vi "Set API Server.vi"(8 "error in (no error)":errorcluster, 11 "API Server":T1) -> (0 "error out":errorcluster)   [LabVIEW 2020, in "GCentral-API.lvlib"]
uses:
  GCentral-API.lvlib
  API Server.ctl
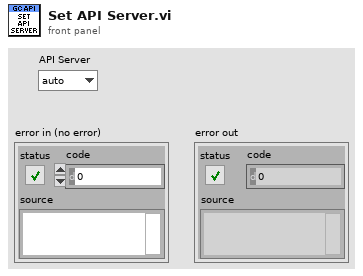
[diagram p1: front panel]
types:
  T1 = typedef "GCentral-API.lvlib/API Server.ctl" = enum16{"auto", "live", "test", "local"}
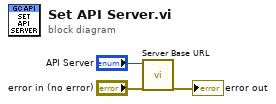
[diagram p0: block diagram]
diagram:
  n1 = call "Server Base URL.vi"("API Server (auto)"="API Server") -> ()  [unwired: 10 in, 1 out]
  "error out" <- "error in (no error)"
